vi "Vision2.vi"() -> ()   [LabVIEW 2017]
uses:
  <vilib>/userdefined/High Color/IMAQdx.ctl
  <vilib>/vision/driver/IMAQdx.llb/IMAQdx Acquisition Mode.ctl
  <vilib>/vision/driver/IMAQdx.llb/IMAQdx Buffer Number Mode.ctl
  <vilib>/vision/driver/NI_Vision_Acquisition_Software.lvlib
panel:
  in  "Session In":T1="cam0"
  out "Image":T2(plugin-control)
  out "Waveform Chart":dbl(graph)
  in  "stop":bool
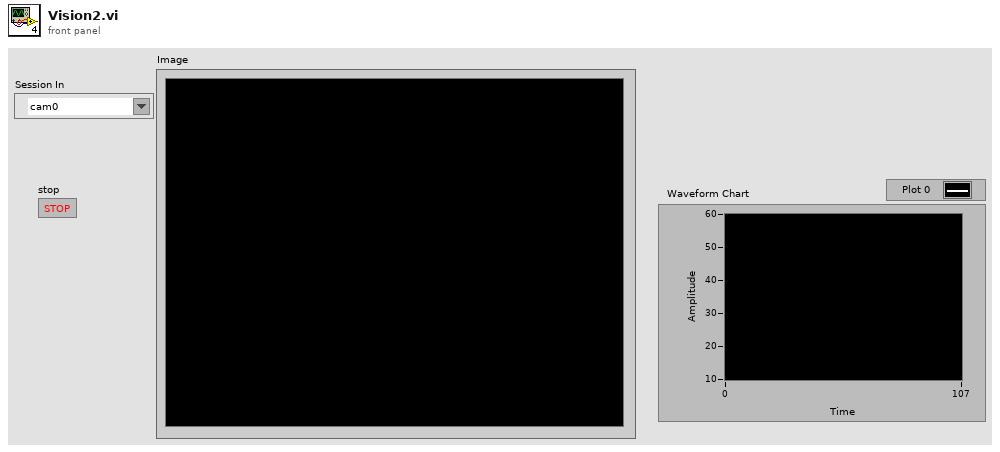
[diagram p1: front panel]
types:
  T1 = typedef "IMAQdx.ctl" = refnum<k21>
  T2 = typedef "IMAQ Image.ctl" = refnum<image>
  T3 = typedef "NI_Vision_Acquisition_Software.lvlib/IMAQdx Acquisition Mode.ctl" = enum32{"One Shot", "Continuous"}
  T4 = typedef "NI_Vision_Acquisition_Software.lvlib/IMAQdx Buffer Number Mode.ctl" = enum32{"Next", "Last", "Buffer Number", "Every", "Last New"}
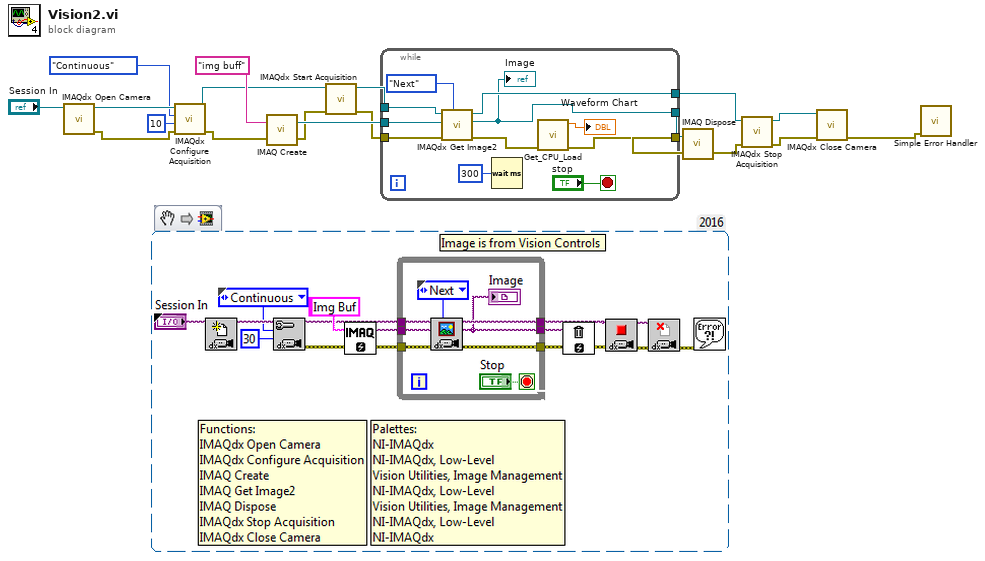
[diagram p0: block diagram]
diagram:
  n1 = call <vilib>:"IMAQdx Open Camera.vi"("Session In"="Session In") -> ("error out"=w14:errorcluster, "Session Out"=w15:T1)  [unwired: 9 in]
  n2 = call <vilib>:"IMAQdx Configure Acquisition.vi"("error in"=w14, "Number of Buffers"=u32 10, "Continuous?"=IMAQdx_Acquisition_Mode."Continuous", "Session In"=w15) -> ("error out"=w18:errorcluster, "Session Out"=w4:T1)  [unwired: 6 in]
  n3 = call "IMAQ Create"("Image Name"="img buff", "error in (no error)"=w18) -> ("New Image"=w16:T2, "error out"=w3:errorcluster)  [unwired: 3 in]
  n4 = call <vilib>:"IMAQdx Start Acquisition.vi"("error in"=w3, "Session In"=w4) -> ("error out"=w2:errorcluster, "Session Out"=w1:T1)  [unwired: 8 in]
  n5 = while {
    tunnel: [w28] -> w13
    tunnel: [w21] -> w12
    tunnel: [w26] -> w11
    tunnel: w1 -> [w25]
    tunnel: w16 -> [w24]
    tunnel: w2 -> [w23]
    stop <- "stop" stop-if-true
    n6 = call <vilib>:"IMAQdx Get Image2.vi"("Buffer Number Mode (Next)"=IMAQdx_Buffer_Number_Mode."Next", "error in"=w23, "Image In"=w24, "Session In"=w25) -> ("error out"=w29:errorcluster, "Image Out"=w21:T2, "Session Out"=w26:T1)  [unwired: 4 in, 1 out]
    "Image" <- w21
    n7 = Wait (ms)(milliseconds to wait=u32 300) -> ()  [unwired: 1 out]
    n8 = call "Get_CPU_Load.vi"("error in (no error)"=w29) -> ("error out"=w28:errorcluster, "Numeric"=→"Waveform Chart":dbl)  [unwired: 9 in]
  }
  n9 = call "IMAQ Dispose"("Image"=w12, "error in (no error)"=w13) -> ("error out"=w10:errorcluster)  [unwired: 4 in]
  n10 = call <vilib>:"IMAQdx Stop Acquisition.vi"("error in"=w10, "Session In"=w11) -> ("error out"=w9:errorcluster, "Session Out"=w8:T1)  [unwired: 8 in]
  n11 = call <vilib>:"IMAQdx Close Camera.vi"("error in"=w9, "Session In"=w8) -> ("error out"=w7:errorcluster)  [unwired: 9 in]
  n12 = call <vilib>:"Simple Error Handler.vi"("error in (no error)"=w7) -> ()  [unwired: 4 in, 5 out]
